vi "ExFileReadNConvertToDatatype.vi"() -> ()   [LabVIEW 2010]
panel:
  in  "Output file name":path
  in  "data type":u32=7 min=1 max=8 step=1
  in  "Full File Name":path
  in  "?":bool
  in  "FileType":u32=67371008
  out "error out":errorcluster
  in  "error in (no error)":errorcluster
  # "File Types:\nSPE = 67371008\nTIF   = 67174400\nPMI  = 67436544"
  # "ExReadFileNconvertToU16.vi\nThis example will read in a file of the\nselected data type and display as u16 frame.\nWhen finished viewing data, make sure to\nuse the STOP button to close the display."
  # "Browse match pattern is set to *.spe.  Modify this if different file type is needed."
  # "This will properly close the image and deallocate memory."
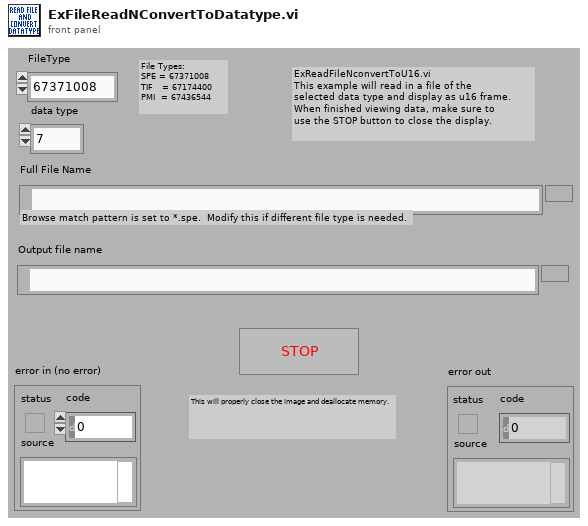
[diagram p1: front panel]
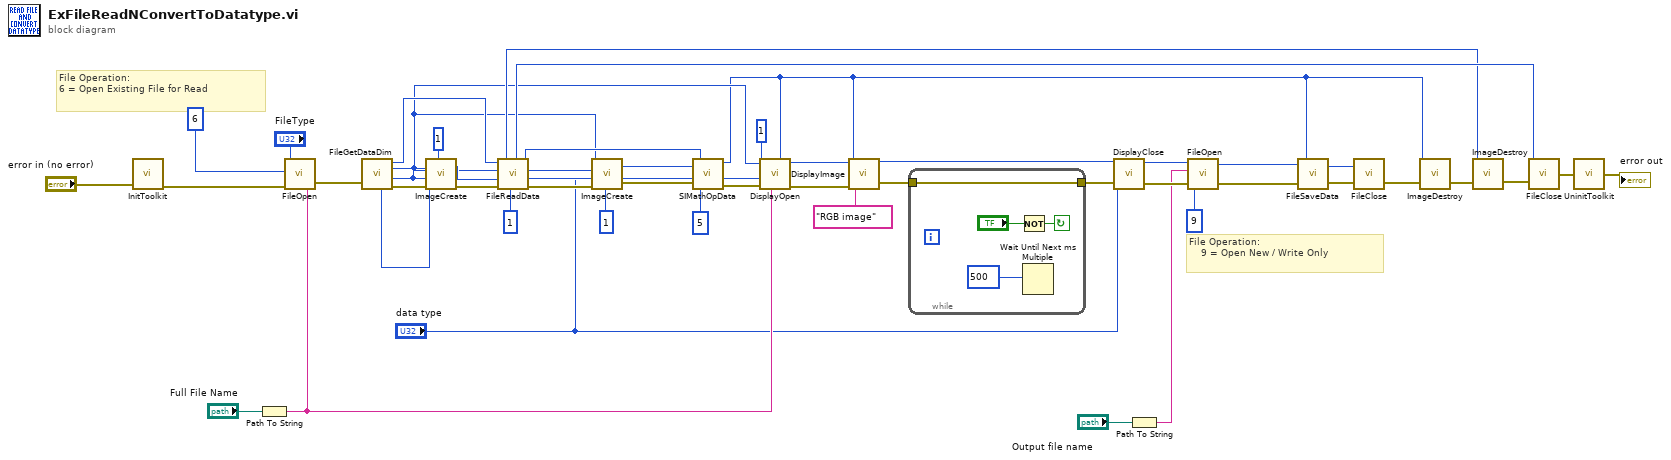
[diagram p0: block diagram]
diagram:
  w33 = 1
  # "File Operation:\n    9 = Open New / Write Only"
  # "File Operation:\n6 = Open Existing File for Read"
  n1 = call <userlib>:"InitToolkit.vi"("error in"="error in (no error)") -> ("error out"=w45:errorcluster)
  n2 = Path To String(path="Full File Name") -> (string=w36:string)
  n3 = call <userlib>:"FileOpen.vi"("error in"=w45, "File Operations"=u32 6 ("File Operation"), "FileName"=w36, "File Type"="FileType") -> ("error out"=w43:errorcluster, "File Handle"=w42:u32)
  n4 = call <userlib>:"FileGetDataDim.vi"("File Handle"=w42, "error in"=w43) -> ("Data Type"=w23:u32, "File Handle"=w35:u32, "X dim"=w6:u32, "Y dim"=w5:u32, "error out"=w20:errorcluster)  [unwired: 1 out]
  n5 = call <userlib>:"ImageCreate.vi"("X dimension"=w6, "Y dimension"=w5, "Data Type"=w23, "error in"=w20, "Number Of Frames"=1) -> ("Image Handle"=w25:u32, "error out"=w34:errorcluster)
  n6 = call <userlib>:"FileReadData.vi"("File Handle"=w35, "Start Frame"=w33, "End Frame"=w33, "error in"=w34, "Image Handle"=w25) -> ("File Handle"=w32:u32, "Image Handle"=w17:u32, "error out"=w21:errorcluster)
  n7 = call <userlib>:"ImageCreate.vi"("X dimension"=w6, "Y dimension"=w5, "Data Type"="data type", "error in"=w21, "Number Of Frames"=1) -> ("Image Handle"=w18:u32, "error out"=w19:errorcluster)
  n8 = call <userlib>:"SIMathOpData.vi"("error in (no error)"=w19, "Operation"=5, "Result Handle"=w18, "Data Handle"=w17) -> ("error out"=w15:errorcluster, "Result Handle"=w4:u32)
  n9 = call <userlib>:"DisplayOpen.vi"("Display Title"=w36, "Image Handle"=w4, "error in"=w15, "Display Height"=w5, "Display Width"=w6, "Display Type"=1) -> ("error out"=w31:errorcluster, "Display Handle"=w30:u32)
  n10 = call <userlib>:"DisplayImage.vi"("error in"=w31, "Title"="RGB image", "Image Handle"=w4, "Display Handle"=w30) -> ("error out"=w24:errorcluster, "Display Handle"=w29:u32)
  n11 = while {
    tunnel: w24 -> [w48]
    tunnel: [w48] -> w9
    stop <- w50 continue-if-true
    n12 = Not(x="?") -> (.not. x?=w50:bool)
    n13 = Wait Until Next ms Multiple(millisecond multiple=500) -> ()  [unwired: 1 out]
  }
  n14 = call <userlib>:"DisplayClose.vi"("error in"=w9, "Display Handle"=w29) -> ("error out"=w8:errorcluster)
  n15 = Path To String(path="Output file name") -> (string=w2:string)
  n16 = call <userlib>:"FileOpen.vi"("error in"=w8, "File Operations"=9, "FileName"=w2, "File Type"="data type") -> ("error out"=w14:errorcluster, "File Handle"=w12:u32)
  n17 = call <userlib>:"FileSaveData.vi"("error in"=w14, "Image Handle"=w4, "File Handle"=w12) -> ("error out"=w13:errorcluster, "File Handle"=w11:u32)
  n18 = call <userlib>:"FileClose.vi"("error in"=w13, "File Handle"=w11) -> ("error out"=w7:errorcluster)
  n19 = call <userlib>:"ImageDestroy.vi"("error in"=w7, "Data handle"=w4) -> ("error out"=w28:errorcluster)
  n20 = call <userlib>:"ImageDestroy.vi"("error in"=w28, "Data handle"=w25) -> ("error out"=w27:errorcluster)
  n21 = call <userlib>:"FileClose.vi"("error in"=w27, "File Handle"=w32) -> ("error out"=w39:errorcluster)
  n22 = call <userlib>:"UninitToolkit.vi"("error in"=w39) -> ("error out"=→"error out":errorcluster)
